vi "AlliGator Remove Duplicated Fit Parameter Constraints.vi"(8 "Error In":errorcluster, 9 "New Constraints in":T1[](array[typedef]) {"Max Value" format="%#.3g"; "Min Value" format="%#.3g"}, 11 "Old Constraints":T1[](array[typedef]) {"Max Value" format="%#.3g"; "Min Value" format="%#.3g"}) -> (0 "Error Out":errorcluster, 1 "Offset Fitted?":bool, 3 "New Constraints out":T1[](array[typedef]) {"Max Value" format="%#.3g"; "Min Value" format="%#.3g"})   [LabVIEW 2021, in "AlliGator Settings.lvlib"]
doc: "Removes any potential duplicate entries in the array of fit parameter constraints."
uses:
  AlliGator Settings.lvlib
  Decay Analysis/Decay Fit/AlliGator Decay Fit Parameter Constraints 2.ctl
  359a0e18-36cc-47c1-bd4d-14aca24d9214.vi
  462271ff-30ec-4d38-93df-9dde4097cd5c.vi
  359a0e18-36cc-47c1-bd4d-14aca24d9214.vi/8dd81a27-1ff4-4680-915d-7458584d3105.vi
  <userlib>/_OpenG.lib/array/array.llb/Sort Array__ogtk.vi
  <userlib>/_OpenG.lib/array/array.llb/Sort 1D Array (I32)__ogtk.vi
  <userlib>/_OpenG.lib/array/array.llb/Reorder Array2__ogtk.vi
  <userlib>/_OpenG.lib/array/array.llb/Reorder 1D Array2 (I32)__ogtk.vi
  <userlib>/_OpenG.lib/array/array.llb/Delete Elements from 1D Array (Variant)__ogtk.vi
  <userlib>/_OpenG.lib/array/array.llb/openg_array.lvlib
  Decay Analysis/Decay Fit/AlliGator Decay Fit.lvlib
  Fits/IRF(X)PSED/Decay Fit Parameters In List.ctl
  Fits/Fits.lvlib
panel:
  # "see the AlliGator License on the block diagram (Ctrl+E or Window:Show Block Diagram)"
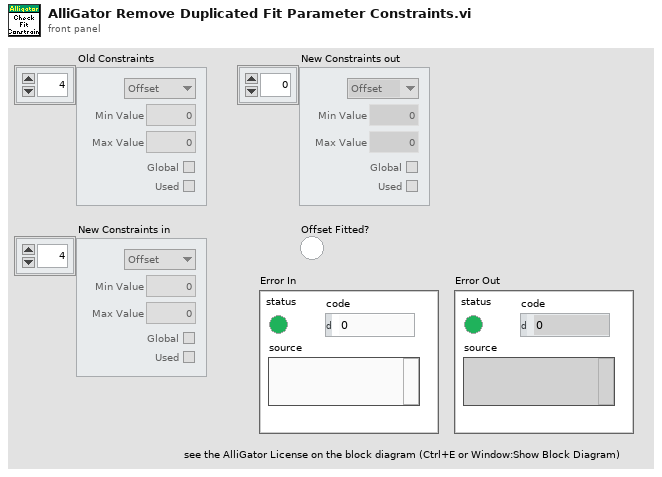
[diagram p1: front panel]
types:
  T1 = typedef "AlliGator Decay Fit.lvlib/AlliGator Decay Fit Parameter Constraints 2.ctl" = cluster{"Fit Parameter":T2, "Min Value":dbl, "Max Value":dbl, "Global":bool, "Used":bool}
  T2 = typedef "Fits.lvlib/Decay Fit Parameters In List.ctl" = enum16{"Offset", "Baseline", "A_1", "tau_1", "A_2", "tau_2"}
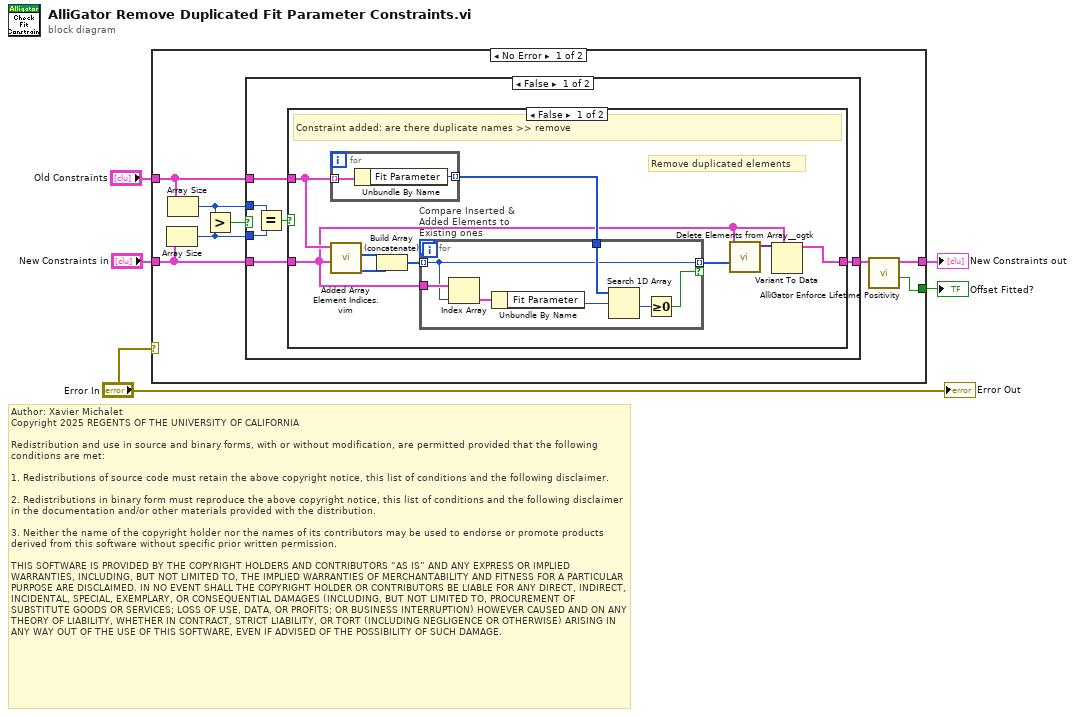
[diagram p0: block diagram]
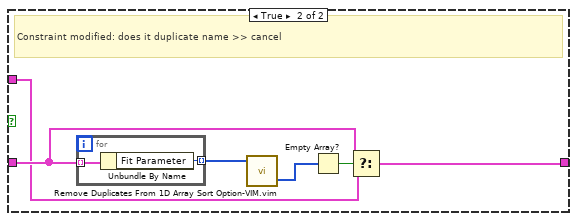
[diagram p2: hidden frame]
diagram:
  # "Author: Xavier Michalet\nCopyright 2025 REGENTS OF THE UNIVERSITY OF CALIFORNIA\n\nRedistribution and use in source and binary forms, with or without modification, are permitted provided that the following conditions are met:\n\n1. Redistributions of source code must retain the above copyright notice, this list of conditions and the following disclaimer.\n\n2. Redistributions in binary form must reproduce the above copyright notice, this list of conditions and the following disclaimer in the documentation and/or other materials provided with the distribution.\n\n3. Neither the name of the copyright holder nor the names of its contributors may be used to endorse or promote products derived from this software without specific prior written permission.\n\nTHIS SOFTWARE IS PROVIDED BY THE COPYRIGHT HOLDERS AND CONTRIBUTORS “AS IS” AND ANY EXPRESS OR IMPLIED WARRANTIES, INCLUDING, BUT NOT LIMITED TO, THE IMPLIED WARRANTIES OF MERCHANTABILITY AND FITNESS FOR A PARTICULAR PURPOSE ARE DISCLAIMED. IN NO EVENT SHALL THE COPYRIGHT HOLDER OR CONTRIBUTORS BE LIABLE FOR ANY DIRECT, INDIRECT, INCIDENTAL, SPECIAL, EXEMPLARY, OR CONSEQUENTIAL DAMAGES (INCLUDING, BUT NOT LIMITED TO, PROCUREMENT OF SUBSTITUTE GOODS OR SERVICES; LOSS OF USE, DATA, OR PROFITS; OR BUSINESS INTERRUPTION) HOWEVER CAUSED AND ON ANY THEORY OF LIABILITY, WHETHER IN CONTRACT, STRICT LIABILITY, OR TORT (INCLUDING NEGLIGENCE OR OTHERWISE) ARISING IN ANY WAY OUT OF THE USE OF THIS SOFTWARE, EVEN IF ADVISED OF THE POSSIBILITY OF SUCH DAMAGE."
  n1 = case shown="No Error" "Error In" {
    tunnel: "New Constraints in" -> [w12 w47]
    tunnel: [w7 w47] -> w4
    tunnel: "Old Constraints" -> [w10 _]
    tunnel: [w6 _] -> w1
    frame No Error {
      n2 = Array Size(array=w12) -> (size(s)=w9:i32)
      n3 = Array Size(array=w10) -> (size(s)=w8:i32)
      n4 = Greater?(x=w8, y=w9) -> (0:w13:bool)
      n5 = case shown="False" w13 {
        tunnel: w12 -> [w15 w46]
        tunnel: [w14 w46] -> w11
        tunnel: w10 -> [w16 _]
        tunnel: w9 -> [w18 _]
        tunnel: w8 -> [w19 _]
        frame False {
          n6 = Equal?(x=w19, y=w18) -> (x = y?=w17:bool)
          n7 = case shown="False" w17 {
            tunnel: w16 -> [w28 w41]
            tunnel: w15 -> [w24 w43]
            tunnel: [w22 w42] -> w14
            frame False {
              # "Remove duplicated elements"
              # "Constraint added: are there duplicate names >> remove"
              n8 = for {
                tunnel: w28 -> [w37] mode=indexing
                tunnel: [w36] -> w26 mode=indexing
                n9 = Unbundle By Name(w37) -> ("Fit Parameter"=w36:T2)
              }
              n10 = call "Added Array Element Indices.vim"("New Array"=w24, "Old Array"=w28) -> ("Appended Element Indices in New Array"=w20:i32[], "Inserted Element Indices in New Array"=w21:i32[])  [unwired: 6 in, 2 out]
              n11 = Build Array (concatenate)(w21, w20) -> (w27:i32[])
              n12 = for "Compare Inserted & Added Elements to Existing ones" {
                tunnel: w27 -> [w30] mode=indexing
                tunnel: w24 -> [w35]
                tunnel: w26 -> [w33]
                tunnel: [w30] -> w25 mode=indexing if=w29
                n13 = Index Array(array=w35, index=w30) -> (element=w34:T1)
                n14 = Unbundle By Name(w34) -> ("Fit Parameter"=w32:T2)
                n15 = Search 1D Array(1D array=w33, element=w32) -> (index of element=w31:i32)  [unwired: 1 in]
                n16 = Greater Or Equal To 0?(x=w31) -> (x >= 0?=w29:bool)
              }
              n17 = call-poly <userlib>:"Delete Elements from Array__ogtk.vi"("indices"=w25, "array"=w24) -> ("array w/ subset deleted"=w23:variant[])  [unwired: 8 in, 1 out]
              n18 = Variant To Data(type=w24, Variant=w23) -> (data=w22:T1[])  [unwired: 1 in, 1 out]
            }
            frame True {
              # "Constraint modified: does it duplicate name >> cancel"
              n19 = for {
                tunnel: w43 -> [w45] mode=indexing
                tunnel: [w44] -> w40 mode=indexing
                n20 = Unbundle By Name(w45) -> ("Fit Parameter"=w44:T2)
              }
              n21 = call "Remove Duplicates From 1D Array Sort Option-VIM.vim"("Input Array"=w40) -> ("Indices of Removed Elements"=w39:i32[])  [unwired: 1 in, 1 out]
              n22 = Empty Array?(array=w39) -> (empty?=w38:bool)
              n23 = Select(t=w43, s=w38, f=w41) -> (s? t:f=w42:T1[])
            }
          }
        }
        frame True {
          # "Constraint deleted: no checks"
        }
      }
      n24 = call "AlliGator Enforce Lifetime Positivity.vi"("Constraints in"=w11) -> ("Offset Fitted"=w6:bool, "Constraints out"=w7:T1[])  [unwired: 9 in]
    }
    frame Error {
    }
  }
  "New Constraints out" <- w4
  "Offset Fitted?" <- w1
  "Error Out" <- "Error In"
